vi "Set Bias Voltage.vi"(8 "error in (no error)":errorcluster, 9 "Channel":i32, 10 "Bias Voltage (V)":dbl, 11 "Example in":refnum<class "Instrument.Template.lvclass">) -> (0 "error out":errorcluster, 3 "Example out":refnum<class "Instrument.Template.lvclass">)   [LabVIEW 2019, in "Instrument.Template.lvclass"]
uses:
  Instrument.Template.lvclass
  C:/Users/patrick/Documents/GitHub/Instrument-Framework/.lvsrc/SMOs/Instrument/Instrument.lvclass
  Typedefs/Instrument.Template.Commands--Enum.ctl
  <userlib>/LevyLab/Levylab Instruments/SMOs/Instrument/Instrument.lvclass/Instrument.ctl
  67792bfe-8e2c-4879-abc2-cb448bcec168.vi
  67792bfe-8e2c-4879-abc2-cb448bcec168.vi/33822cc9-4fa3-4844-9d01-3e29f4ba69c9.vi
  67792bfe-8e2c-4879-abc2-cb448bcec168.vi/4c337d88-2c90-4ecf-8ab5-bec3fe174136.vi
  <userlib>/LevyLab/Levylab Instruments/SMOs/Instrument/API/Send and Receive.vi
  67792bfe-8e2c-4879-abc2-cb448bcec168.vi/4c337d88-2c90-4ecf-8ab5-bec3fe174136.vi/809e0d3f-8fa7-4b0f-93ea-879f94b19e70.vi
  67792bfe-8e2c-4879-abc2-cb448bcec168.vi/4c337d88-2c90-4ecf-8ab5-bec3fe174136.vi/6df4db00-b645-4072-83a9-419f610704e0.vi
  <userlib>/LevyLab/Levylab Instruments/SMOs/Instrument/API/Open.vi
  <userlib>/LevyLab/Levylab Instruments/SMOs/RemoteControl/API/Send and Receive.vi
  <vilib>/JDP Science/JSONtext/JSON text to Variant.vi
  <userlib>/LevyLab/Levylab Instruments/SMOs/Instrument/API/Close.vi
  <vilib>/JDP Science/JSONtext/LVClass Serializer/JSONtext LVClass Serializer.lvclass
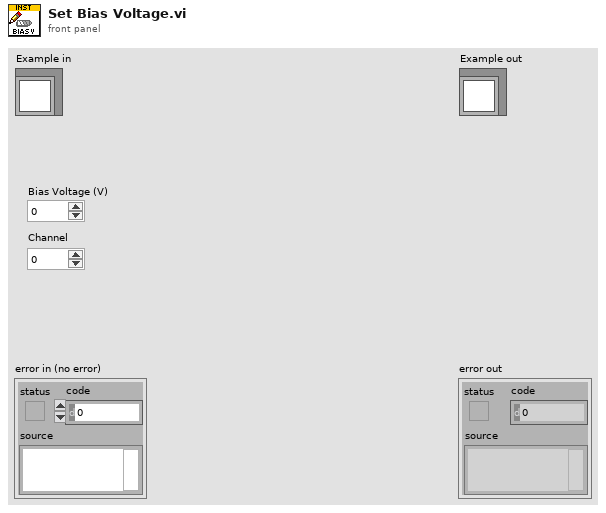
[diagram p1: front panel]
types:
  T1 = typedef "Instrument.Template.lvclass/Instrument.Template.Commands--Enum.ctl" = enum16{"command0", "command1", "command2"}
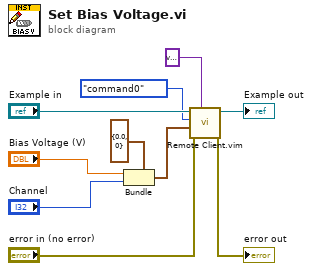
[diagram p0: block diagram]
diagram:
  n1 = Bundle(cluster=cluster{"Bias Voltage (V)":dbl, "Channel":i32} {"Bias Voltage (V)"=0.0, "Channel"=0} ("output cluster"), "Bias Voltage (V)"="Bias Voltage (V)", "Channel"="Channel") -> (w3:cluster{"Bias Voltage (V)":dbl, "Channel":i32})
  n2 = call "Remote Client.vim"("Data Out type"=variant, "error in (no error)"="error in (no error)", "params"=w3, "method"=Instrument.Template.Commands--Enum."command0" ("Commands"), "Instrument in"="Example in") -> ("error out"=→"error out":errorcluster, "Instrument out"=→"Example out":refnum<class "Instrument.Template.lvclass">)  [unwired: 3 in, 2 out]
